vi "ep_Get Predefined Property Names.vi"() -> (3 "pre-defined property names":string[](array[string]))   [LabVIEW 2011, in "NI_EP_COMTRADE.lvlib"]
uses:
  <vilib>/addons/Electrical Power/File IO/NI_EP_COMTRADE.lvlib
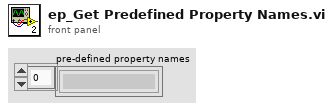
[diagram p1: front panel]
types:
  T1 = typedef "dataModel.ctl" = cluster{"typeDef":T2, "Properties":T3[]}
  T2 = typedef "usiTypeDef.ctl" = cluster{"name":string, "baseName":string, "abstract":bool}
  T3 = typedef "usiPropDef.ctl" = cluster{"name":string, "baseName":string, "refDataType":string, "dimensions":i32, "type":i32, "user defined":bool, "enumStrings":string[], "usiDataType":T4, "specialProp":T5, "Property Source":string, "index":i32}
  T4 = typedef "usiDataType.ctl" = enum16{"eNoTypeUsi", "eInt8Usi", "eInt16Usi", "eInt32Usi", "eInt64Usi", "eUInt8Usi", "eUInt16Usi", "eUInt32Usi", "eUInt64Usi", "eFloat32Usi", "eFloat64Usi", "- 0", "- 1", "- 2", "- 3", "- 4", "- 5", "- 6", "- 7", "- 8", "- 9", "eString8Usi", "eString16Usi", "eStringUsi", "eEnumUsi", "- 10", "- 11", "- 12", "- 13", "- 14", "eTimeUsi", "- 15", "- 16", "- 17", "- 18", "- 19", "- 20", "- 21", "- 22", "- 23", "eInstanceUsi", "eStoreUsi"}
  T5 = typedef "specialProperties.ctl" = enum16{"<Default>", "Channel Values", "AppendReplace", "ChannelFlags", "ValueFlags", "ImplicitExplicit", "InsertIndex", "ValuesCount", "ComparisonOperator", "Cluster", "DAQmx Channel"}
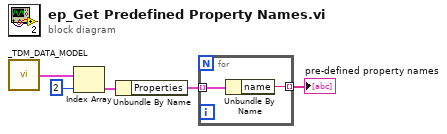
[diagram p0: block diagram]
diagram:
  n1 = call <vilib>:"_TDM_DATA_MODEL.vi"() -> ("objectDefinition"=w5:T1[])
  n2 = Index Array(array=w5, index=2) -> (element=w3:T1)
  n3 = Unbundle By Name(w3) -> ("Properties"=w2:T3[])
  n4 = for {
    tunnel: w2 -> [w7] mode=indexing
    tunnel: [w6] -> w1 mode=indexing
    n5 = Unbundle By Name(w7) -> ("name"=w6:string)
  }
  "pre-defined property names" <- w1
